vi "Query with Scalar Double Result.vi"(8 "error in (no error)":errorcluster, 10 "Query string":string, 11 "mysql in":refnum<class "mysql.lvclass">) -> (0 "error out":errorcluster, 2 "Result":dbl, 3 "mysql out":refnum<class "mysql.lvclass">)   [LabVIEW 2020, in "mysql.lvlib" / "mysql.lvclass"]
uses:
  mysql.lvclass
  c2d378ea-a95f-4d51-af68-4e073f8d7d79.vi
  c2d378ea-a95f-4d51-af68-4e073f8d7d79.vi/3741052b-39a7-42bd-9ec1-f8d2ac120a9d.vi
  private/Mysql command.vi
  private/Mysql data reader Scalar double.vi
  private/ping connection and reopen if needed.vi
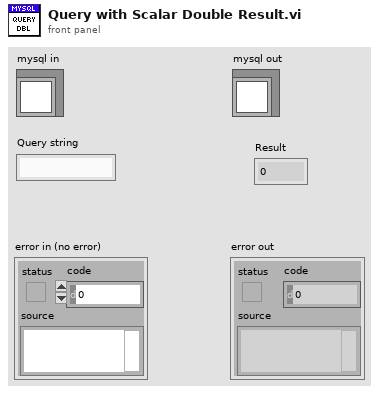
[diagram p1: front panel]
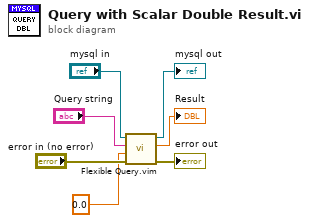
[diagram p0: block diagram]
diagram:
  n1 = call "Flexible Query.vim"("error in (no error)"="error in (no error)", "Type in"=0.0 ("Result 2"), "Query string"="Query string", "mysql in"="mysql in") -> ("error out"=→"error out":errorcluster, "Result"=→"Result":dbl, "mysql out"=→"mysql out":refnum<class "mysql.lvclass">)  [unwired: 5 in]
